vi "oldEnemyTeamToOOEnemyTeam.vi"(5 "Side":enum16{"Esquerdo", "Direito"}(ring), 7 "Team":enum16{"Azul", "Amarelo"}(ring), 8 "error in (no error)":errorcluster, 10 "enemy_robots":T1[](array[typedef]), 11 "Enemy in":refnum<class "Enemy.lvclass">) -> (0 "error out":errorcluster, 3 "Enemy out":refnum<class "Enemy.lvclass">)   [LabVIEW 2020, in "Enemy.lvclass"]
uses:
  Enemy.lvclass
  C:/RoboIME/SSL_AI/Team_class/Team.lvclass
  Robot_class/Robot.lvclass
  C:/RoboIME/SSL_AI/Object_class/Object.lvclass
  Vision_class/Old vision/Controls/AI Robot.ctl
  Vision_class/Old vision/Controls/Functions Enum.ctl
  Controls/estimatives.ctl
  Vision_class/Old vision/Controls/AttackerStates.ctl
  Vision_class/Old vision/Controls/PathDests.ctl
  Vision_class/Old vision/Controls/PathDest.ctl
  Game_class/Navigation/VSSNavigation/VSSAttackerStates.ctl
  Robot_class/robotKickToStates.ctl
  Robot_class/roles.ctl
  Team_class/Team.lvclass/Team.ctl
  Object_class/Object.lvclass/Object.ctl
  Robot_class/Robot.lvclass/Robot.ctl
  Object_class/Write x.vi
  Object_class/Write y.vi
  Robot_class/Write orientation.vi
  Robot_class/Write id.vi
  Robot_class/Write est_v_tang.vi
  Robot_class/Write est_v_norm.vi
  Robot_class/Write est_v_ang.vi
  Object_class/Write pos_est_x.vi
  Object_class/Write pos_est_y.vi
  Team_class/Read RobotRef.vi
  Team_class/Write RobotRef.vi
panel:
  in  "Robot":refnum<class "Robot.lvclass">
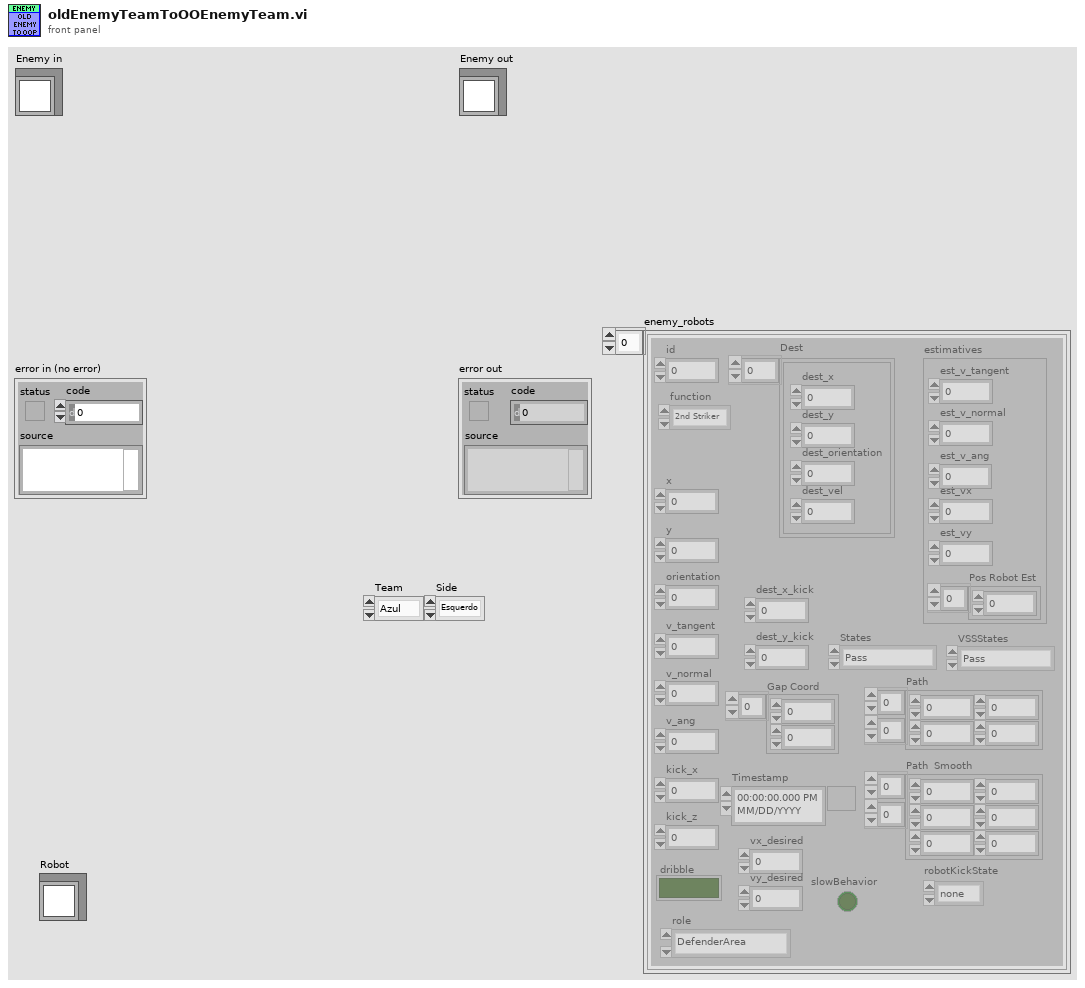
[diagram p1: front panel]
types:
  T1 = typedef "AI Robot.ctl" = cluster{"id":u32, "function":T2, "x":dbl, "y":dbl, "orientation":dbl, "v_tangent":dbl, "v_normal":dbl, "v_ang":dbl, "kick_x":dbl, "kick_z":dbl, "dribble":bool, "Timestamp":timestamp, "estimatives":T3, "dest_x_kick":dbl, "dest_y_kick":dbl, "Gap Coord":dbl[], "States":T4, "Path ":dbl[][], "Path  Smooth":dbl[][], "Dest":T5, "vx_desired":dbl, "vy_desired":dbl, "slowBehavior":bool, "VSSStates":T7, "robotKickState":T8, "role":T9}
  T2 = typedef "Functions Enum.ctl" = enum16{"2nd Striker", "Attacker", "Goalie", "Defender", "Striker", "Goto 0", "Dummy", "Kicker", "ZigZag 0", "ZigZag 1", "ZigZag 2", "ZigZag 3", "ZigZag 4", "ZigZag 5", "ZigZag 6", "ZigZag 7", "ZigZag 8", ""}
  T3 = typedef "estimatives.ctl" = cluster{"est_v_tangent":dbl, "est_v_normal":dbl, "est_vx":dbl, "est_vy":dbl, "Pos Robot Est":dbl[], "est_v_ang":dbl}
  T4 = typedef "AttackerStates.ctl" = enum16{"Pass", "GoToTangent", "BallGetting", "GoToKick", ""}
  T5 = typedef "PathDests.ctl" = T6[]
  T6 = typedef "PathDest.ctl" = cluster{"dest_x":dbl, "dest_y":dbl, "dest_orientation":dbl, "dest_vel":dbl}
  T7 = typedef "VSSAttackerStates.ctl" = enum16{"Pass", "GoToTangent", "BallGetting", "GoToKick", "Rotate anti-clockwise", "Rotate Clockwise", ""}
  T8 = typedef "robotKickToStates.ctl" = enum16{"shootFromDirect", "avoidCollideBall", "goToBackBall", "none", "walk", "turn", "oldKickToShoot", "oldKickToGoToBackBall", "shoot"}
  T9 = typedef "roles.ctl" = enum16{"SimpleBallPlacement", "BallPlacementAllyPasser", "BallPlacementAllyReceiver", "BallPlacementEnemy", "5Robots5th", "PassBestReceiver", "5Robots4th", "5Robots3rd", "5Robots2nd", "5Robots1st", "PassBestRobot", "WaitPass", "ABCThirdKicker", "ABCFirstKicker", "ABCSecondKicker", "Tabler", "TableFinalizer", "PrepareRollToPassRoller", "PrepareRollToPassReceiver", "SimplePassRoll", "SimplePassRollReceiver", "PenaltyDefense", "PreparePassReceiver 2", "PreparePassReceiver 1", "PassObserver", "Timeout", "Goto", "ZigZag", "None", "BallOutOfField", "DefenderArea", "Duelist", "AttackerStop", "FollowAttacker", "KeeperRole", "KickPenalty", "AttackerAimGoal", "AttackerBlock", "Marker", "Halt", "Shoot", "PassKicker", "PassReceiver", "TestRole", "PenaltyAttacker"}
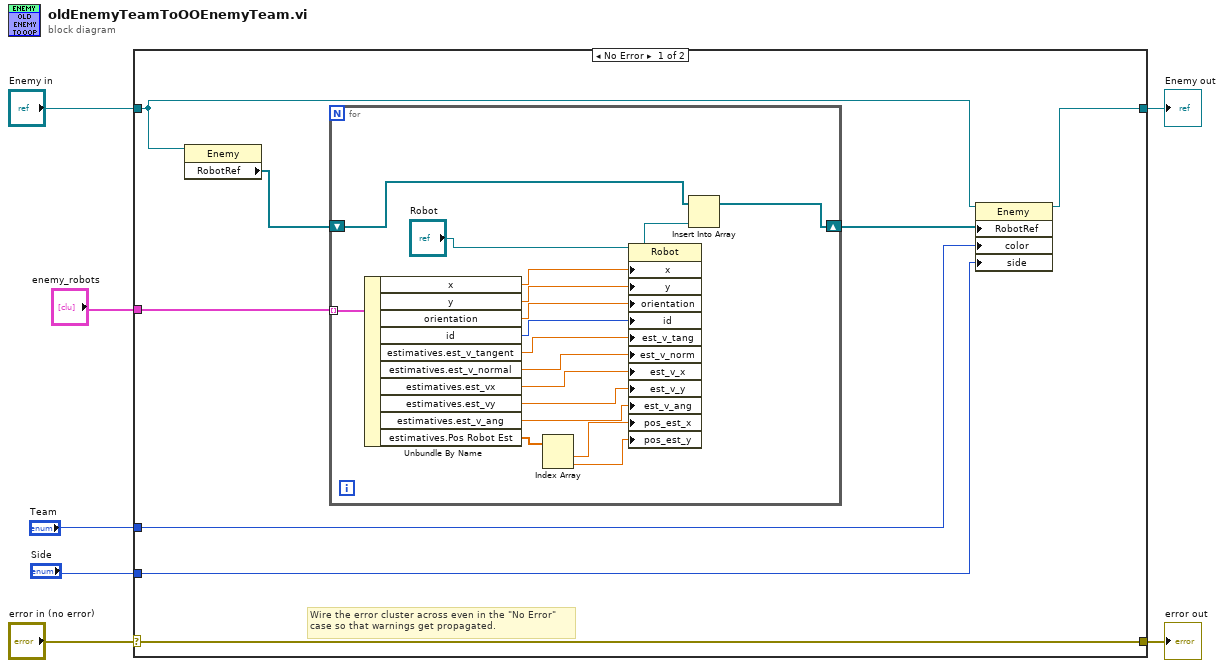
[diagram p0: block diagram]
diagram:
  n1 = case shown="No Error" "error in (no error)" {
    selector: "error in (no error)" -> [w15 w34]
    tunnel: [w15 w34] -> w6
    tunnel: [w12 w33] -> w4
    tunnel: "Enemy in" -> [w10 w33]
    tunnel: "enemy_robots" -> [w11 _]
    tunnel: "Team" -> [w14 _]
    tunnel: "Side" -> [w13 _]
    frame No Error {
      # "Wire the error cluster across even in the \"No Error\"\ncase so that warnings get propagated."
      n2 = property class="Enemy"(reference=w10) -> ("RobotRef"=w9:refnum<class "Robot.lvclass">[])  [unwired: 1 in, 2 out]
      n3 = for {
        shift-right: [w30] -> w8
        shift-left: w9 -> [w28]
        tunnel: w11 -> [w29] mode=indexing
        n4 = Unbundle By Name(w29) -> ("x"=w27:dbl, "y"=w26:dbl, "orientation"=w25:dbl, "id"=w24:u32, "estimatives.est_v_tangent"=w23:dbl, "estimatives.est_v_normal"=w22:dbl, "estimatives.est_vx"=w21:dbl, "estimatives.est_vy"=w20:dbl, "estimatives.est_v_ang"=w19:dbl, "estimatives.Pos Robot Est"=w18:dbl[])
        n5 = Index Array(array=w18) -> (element #1=w17:dbl, element #2=w16:dbl)  [unwired: 2 in]
        n6 = property class="Robot"(reference="Robot", "x"=w27, "y"=w26, "orientation"=w25, "id"=w24, "est_v_tang"=w23, "est_v_norm"=w22, "est_v_x"=w21, "est_v_y"=w20, "est_v_ang"=w19, "pos_est_x"=w17, "pos_est_y"=w16) -> (reference out=w31:refnum<class "Robot.lvclass">)  [unwired: 1 in, 1 out]
        n7 = Insert Into Array(array=w28, new element=w31) -> (w30:refnum<class "Robot.lvclass">[])  [unwired: 1 in]
      }
      n8 = property class="Enemy"(reference=w10, "RobotRef"=w8, "color"=w14, "side"=w13) -> (reference out=w12:refnum<class "Enemy.lvclass">)  [unwired: 1 in, 1 out]
    }
    frame Error {
    }
  }
  "error out" <- w6
  "Enemy out" <- w4
